vi "Actor Core.vi"(8 "error in":errorcluster, 11 "Generic Prompt in":refnum<class "Generic Prompt.lvclass">) -> (0 "Error Out":errorcluster, 3 "Actor out":refnum<class "Actor.lvclass">)   [LabVIEW 2014, in "Generic Prompt.lvlib" / "Generic Prompt.lvclass"]
doc: "(<B>Filename</B>: Actor Framework.lvlib:Actor.lvclass:Actor Core.vi)\n\nReceives messages to the actor, reacts to them, and initiates any error handling that may shut the actor down.\n\nDescendant classes may override this VI to append parallel tasks for the actor to complete while it handles messages. Overrides use the Call Parent Method node."
uses:
  Generic Prompt.lvclass
  <vilib>/ActorFramework/Actor/Actor.lvclass
  SetUp VIs/Instrument Finder/Instrument Finder.lvclass
  Subpanel Insertion/Subpanel Inserter.lvclass
  <vilib>/event_ctls.llb/eventsource.ctl
  <vilib>/event_ctls.llb/lveventtype.ctl
  <vilib>/ActorFramework/Message Enqueuer/Message Enqueuer.lvclass
  <vilib>/ActorFramework/Message Enqueuer/Message Enqueuer.lvclass/Message Enqueuer.ctl
  <vilib>/ActorFramework/Actor/Actor.lvclass/Actor.ctl
  Subpanel Inserter Messages/Insert Into Subpanel Msg/Insert Into Subpanel Msg.lvclass/Insert Into Subpanel Msg.ctl
  <vilib>/ActorFramework/Message Enqueuer/Message Priority.ctl
  New Session Class/New Session.lvclass
  <vilib>/ActorFramework/Message Enqueuer/Enqueue.vi
  <vilib>/ActorFramework/Message Enqueuer/Init from Existing Queue.vi
  <vilib>/ActorFramework/Message Priority Queue/Priority Enqueue.vi
  Subpanel Inserter Messages/Insert Into Subpanel Msg/Insert Into Subpanel Msg.lvclass
  <vilib>/ActorFramework/Stop Msg/Stop Msg.lvclass
  <vilib>/MGI/Monitored Actor/Actor/Monitored Actor.lvclass
panel:
  out "array address size":i32
  out "class name":string
  out "error out 4":errorcluster
  out "error out 3":errorcluster
  in  "cancel kid":bool
  out "Array of addresses":refnum<class "Message Enqueuer.lvclass">[](array[class])
  out "NewVal":bool
  out "OldVal":bool
  out "Time":u32
  out "Type":T1=enum."Value Change"
  out "Source":T2 items=["LabVIEW UI"=0, "ActiveX"=1, "User Event"=25]
  out "stopper":bool
  out "Array 2":string[](array[string])
  out "error out 2":errorcluster
  out "error out":errorcluster
  out "i- main":i32
  out "list of class":string[](array[string])
  out "Array Size":i32
  out "array size = counter? (next)":bool
  out "child to get":i32
  out "New Session SetUp is ON?":bool
  out "VI Name":string
  out "x = 0?":bool
  out "stop?":bool
  out "counter":i32
  out "i":i32
  in  "Array":refnum<class "Subpanel Inserter.lvclass">[](array[class])
  in  "SetUp VIs.lvlib:Instrument Finder.lvclass":refnum<class "Instrument Finder.lvclass">
  in  "Previous Button":bool
  in  "Next Button":bool
  in  "Stop Button":bool
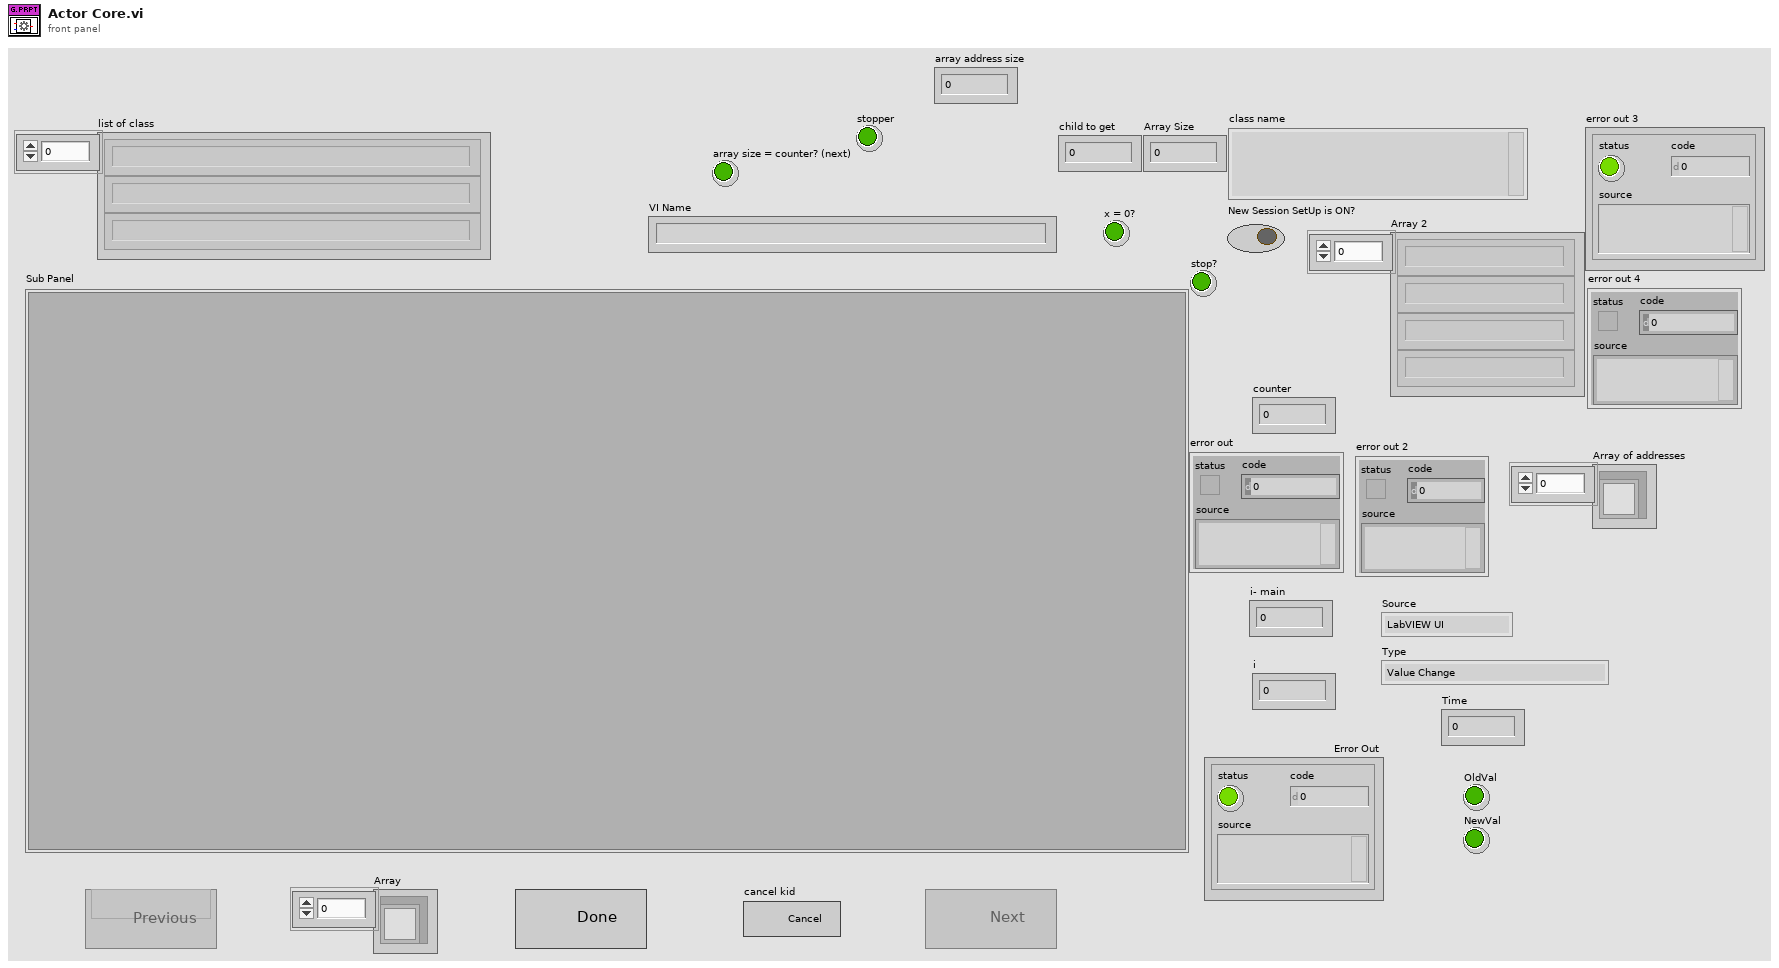
[diagram p1: front panel]
types:
  T1 = typedef "lveventtype.ctl" = enum32{"Null", "Timeout", "Annotation Menu Selection", "Annotation Menu Selection?", "App Instance Close", "App Instance Close?", "Autoscale Range Change", "Bookmark Info Change", "Cell Edit", "Cell Edit?", "Cursor Grab", "Cursor Grab?", "Cursor Menu Selection", "Cursor Menu Selection?", "Cursor Move", "Cursor Release", "Data Change", "Direction Change", "Display State Change", "Drag Ended", "Drag Enter", "Drag Leave", "Drag Over", "Drag Source Update", "Drag Starting", "Drag Starting?", "Drop", "Exec State Change", "Key Down", "Key Down?", "Key Repeat", "Key Repeat?", "Key Up", "Listbox Double Click", "Menu Activation?", "Menu Selection (App)", "Menu Selection? (App)", "Menu Selection (User)", "Mouse Down", "Mouse Down?", "Mouse Enter", "Mouse Leave", "Mouse Move", "Mouse Up", "Mouse Wheel", "NI Security User Change (App)", "Pane Size", "Panel Close", "Panel Close?", "Panel Resize", "Plot Attribute Change", "Scale Range Change", "Shortcut Menu Activation?", "Shortcut Menu Selection (App)", "Shortcut Menu Selection? (App)", "Shortcut Menu Selection (User)", "Tree Double Click", "Tree Drag", "Tree Drag?", "Tree Drop", "Tree Drop?", "Tree Item Close", "Tree Item Close?", "Tree Item Open", "Tree Item Open?", "User Event", "Value Change"}
  T2 = typedef "eventsource.ctl" = u32
  T3 = enum8{"Enabled", "Disabled", "Disabled and Grayed Out"}
  T4 = typedef "Actor Framework.lvlib/Message Enqueuer.lvclass/Message Priority.ctl" = enum16{"Low", "Normal", "High"}
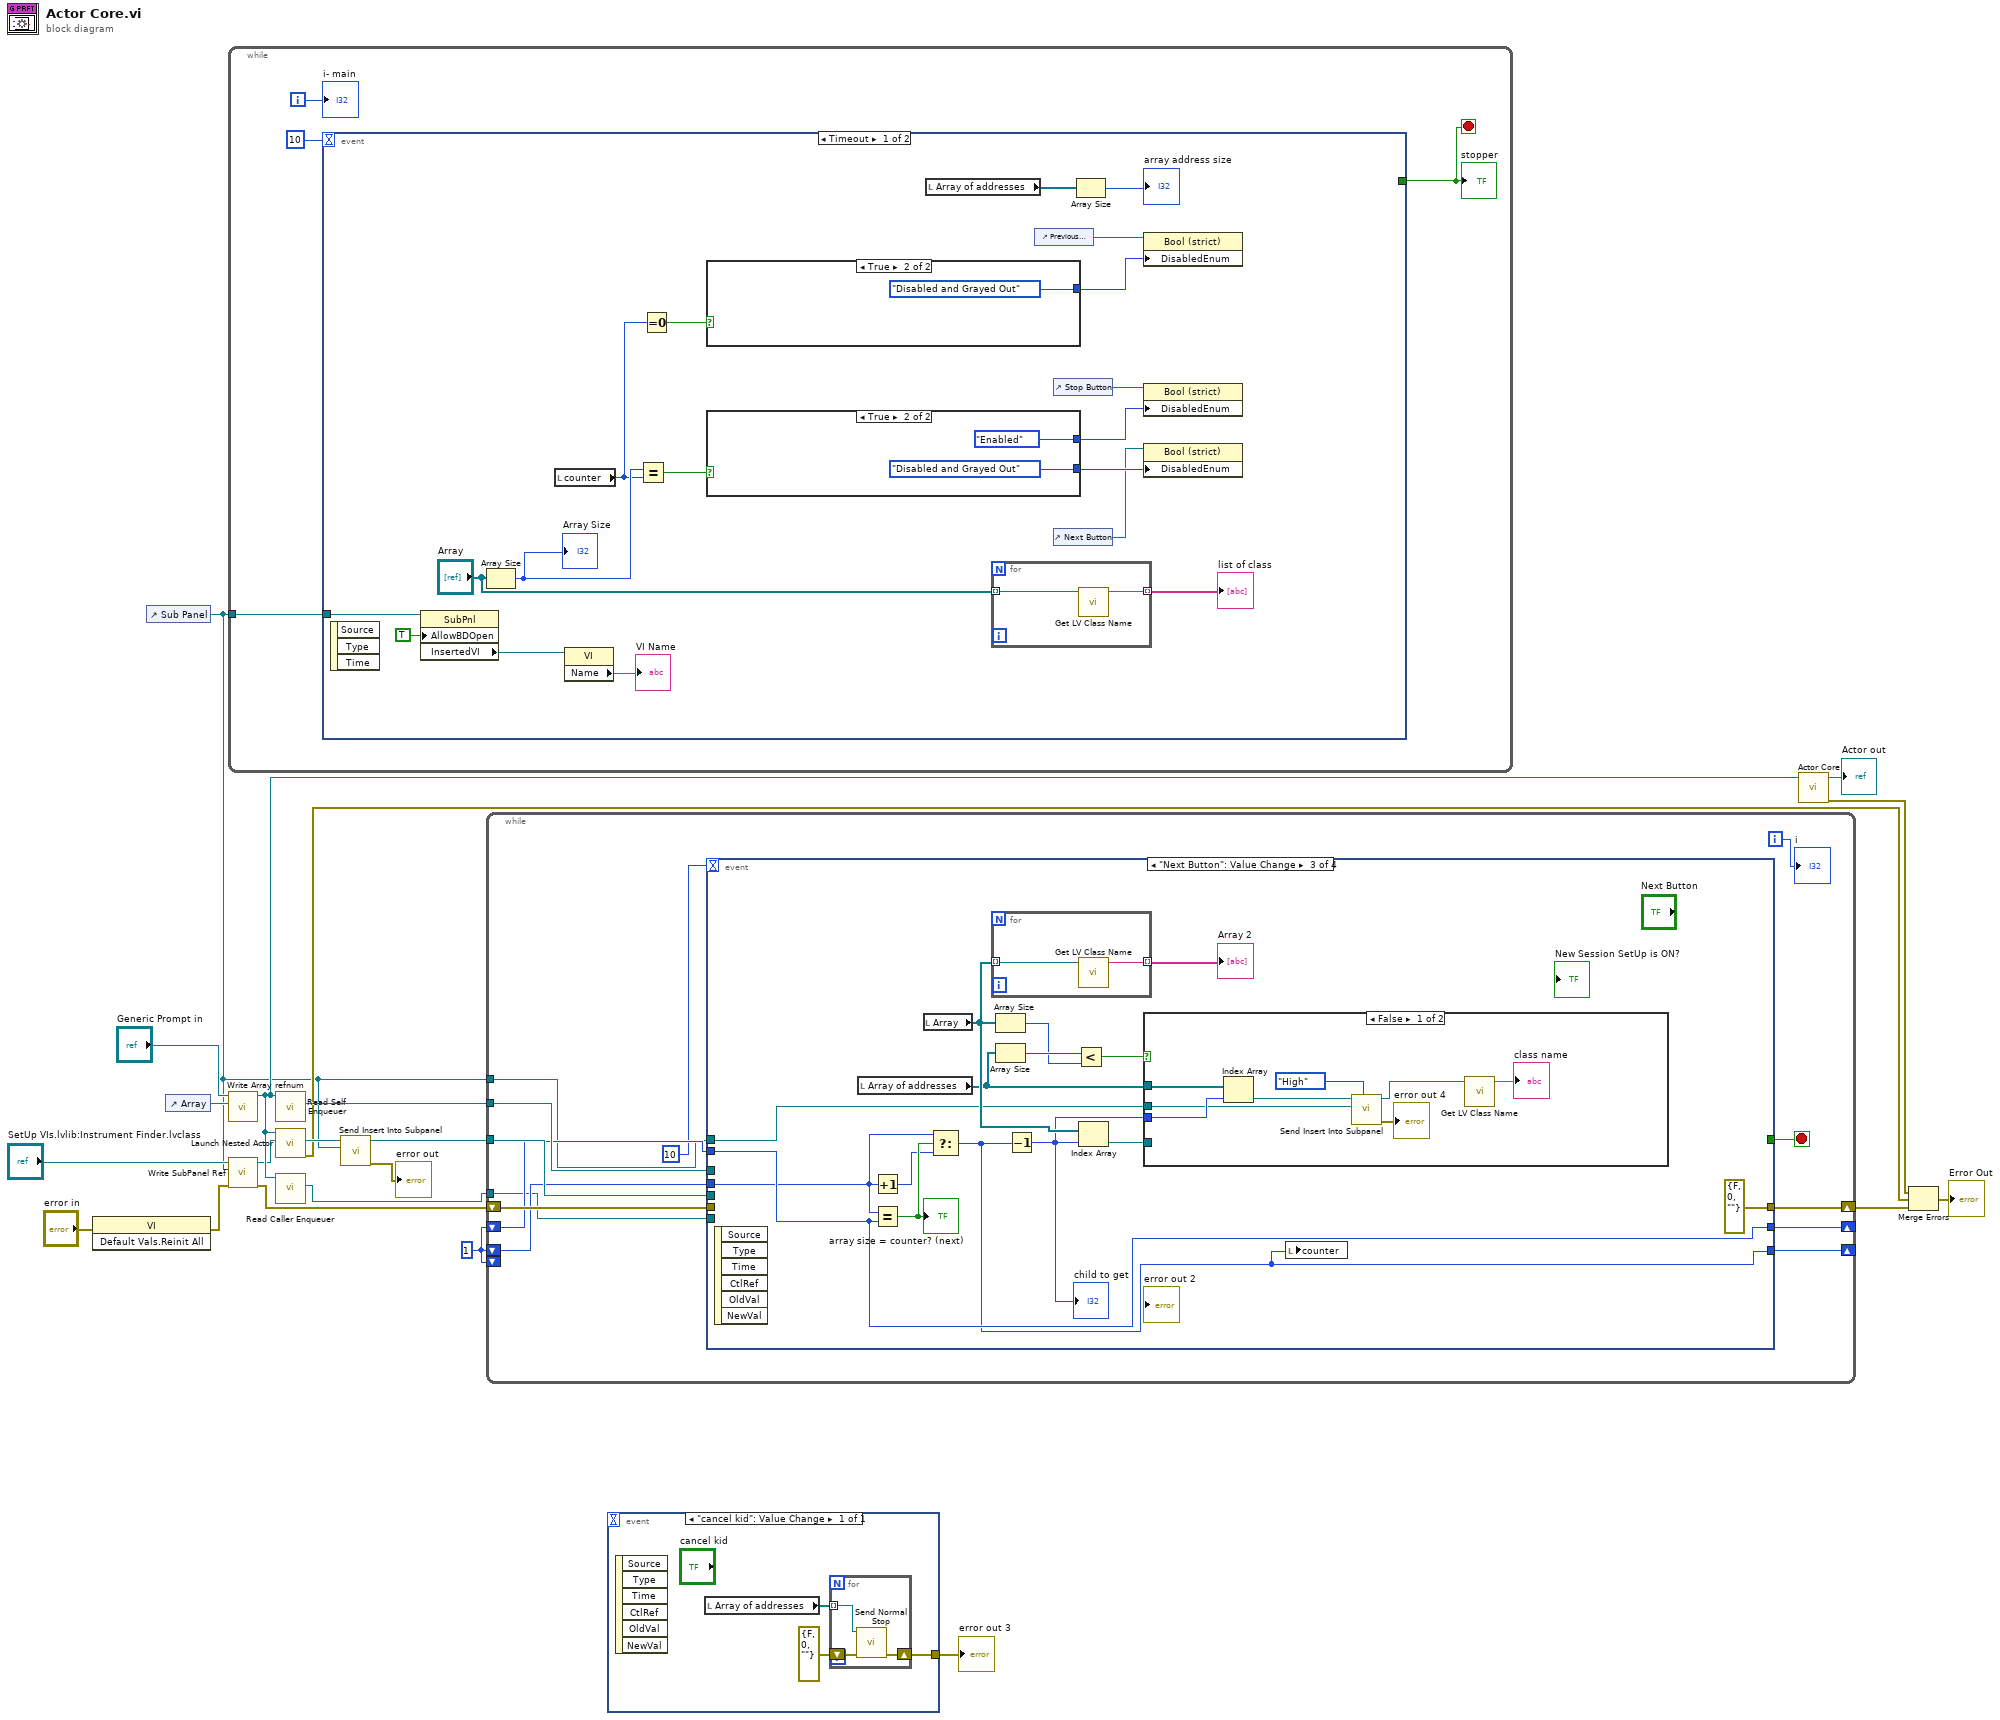
[diagram p0: block diagram]
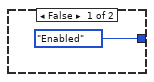
[diagram p2: hidden frame]
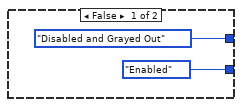
[diagram p3: hidden frame]
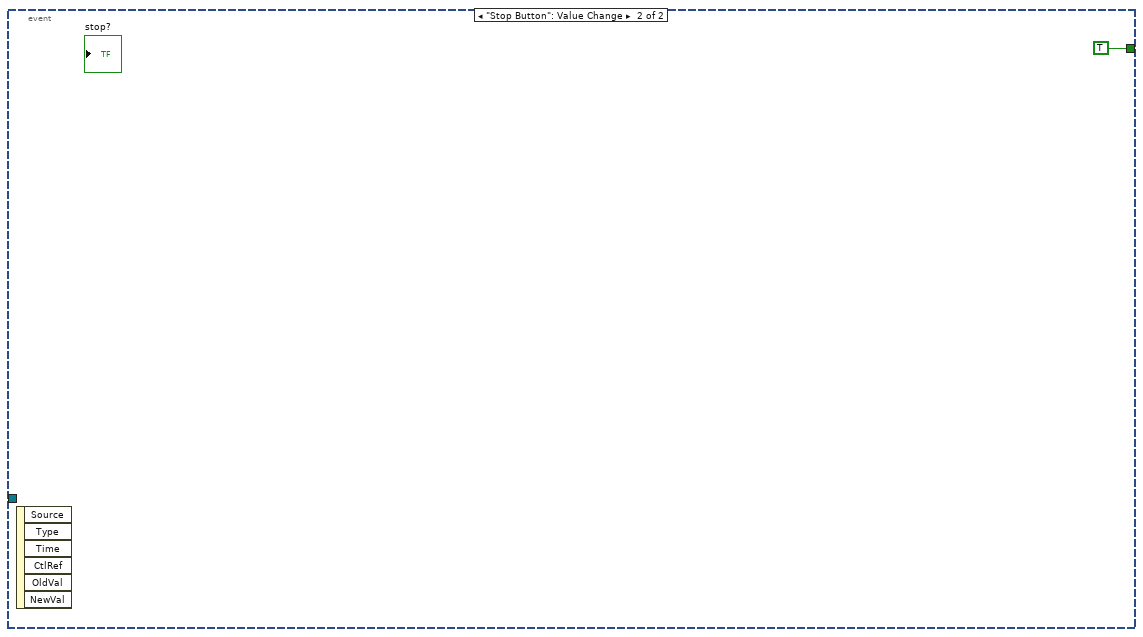
[diagram p4: hidden frame]
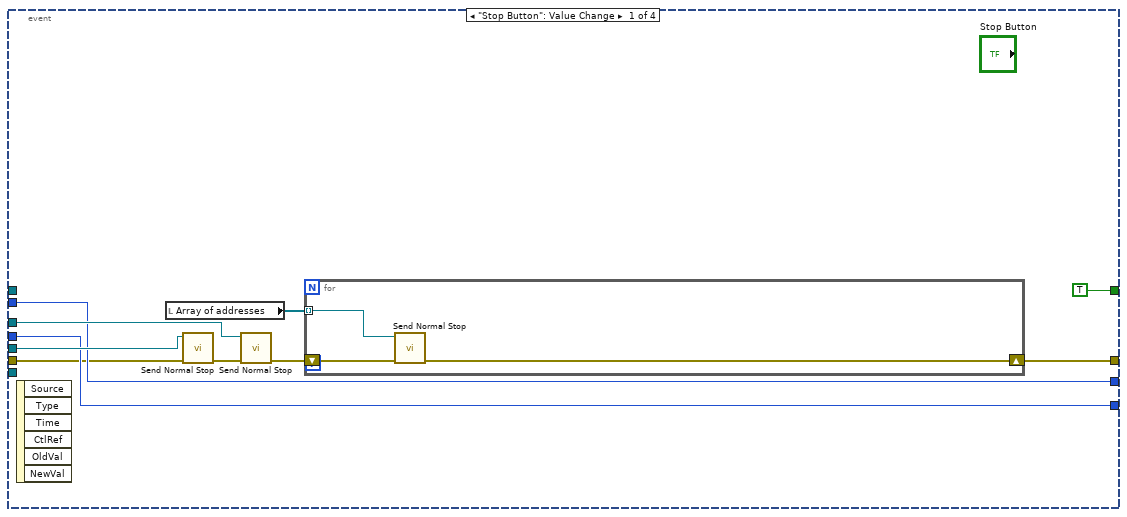
[diagram p5: hidden frame]
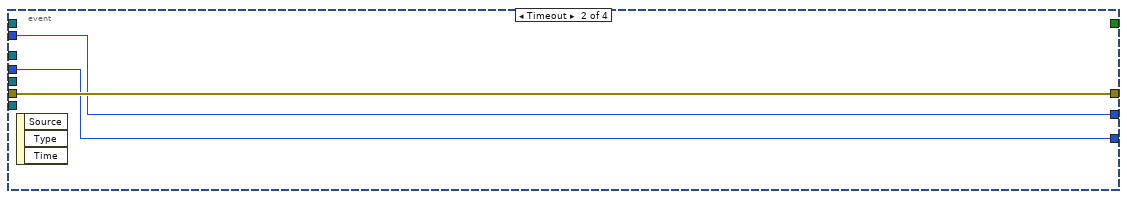
[diagram p6: hidden frame]
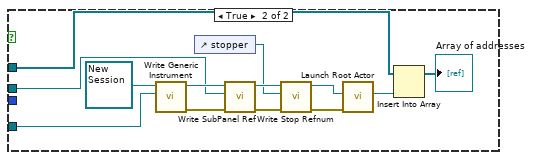
[diagram p7: hidden frame]
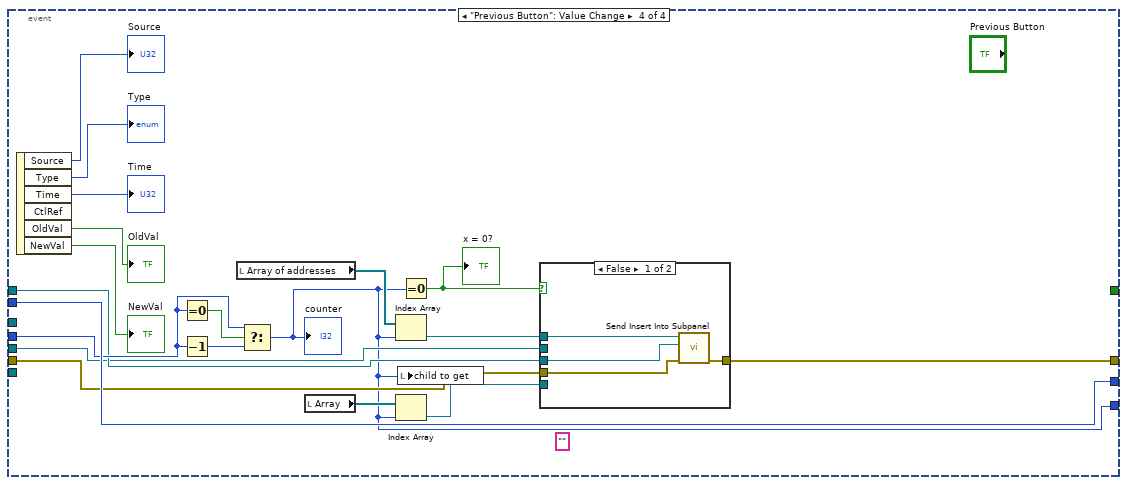
[diagram p8: hidden frame]
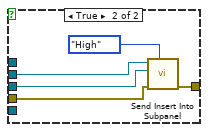
[diagram p9: hidden frame]
diagram:
  w17 = 1
  n1 = invoke class="VI" method="Default Vals.Reinit All"(error in="error in") -> (error out=w19:errorcluster)  [unwired: 2 in, 2 out]
  n2 = control-ref of="Sub Panel"() -> (w3:refnum<vi>)
  n3 = control-ref of="Array"() -> (w11:refnum<vi>)
  n4 = while {
    tunnel: w3 -> [w24]
    i -> [w22]
    stop <- w25 stop-if-true
    n5 = event shown="[0] Timeout" {
      selector: _ -> [_ _]
      dyn-events: _ -> [_ _]
      timeout: 10 -> [_ _]
      tunnel: [_ TRUE] -> w25
      tunnel: w24 -> [w35 _]
      event Timeout {
        n6 = event-data() -> ()  [unwired: 1 in, 3 out]
        n7 = property class="SubPnl"(reference=w35, "AllowBDOpen"=TRUE ("Allow User to Open Diagram")) -> ("InsertedVI"=w37:refnum<vi>)  [unwired: 1 in, 2 out]
        n8 = Array Size(array="Array") -> (size(s)=w31:i32)
        "Array Size" <- w31
        n9 = local read "counter"() -> (w28:i32)
        n10 = property class="VI"(reference=w37) -> ("Name"=→"VI Name":string)  [unwired: 1 in, 2 out]
        n11 = Equal?(x=w31, y=w28) -> (x = y?=w43:bool)
        n12 = Equal To 0?(x=w28) -> (x = 0?=w40:bool)
        n13 = case shown="True" w40 {
          tunnel: [T3."Enabled" ("Disabled") T3."Disabled and Grayed Out" ("Disabled")] -> w41
          frame False {
          }
          frame True {
          }
        }
        n14 = case shown="True" w43 {
          tunnel: [T3."Enabled" ("Disabled") T3."Disabled and Grayed Out" ("Disabled")] -> w42
          tunnel: [T3."Disabled and Grayed Out" ("Disabled") T3."Enabled" ("Disabled")] -> w39
          frame False {
          }
          frame True {
          }
        }
        n15 = local read "Array of addresses"() -> (w27:refnum<class "Message Enqueuer.lvclass">[])
        n16 = for {
          tunnel: "Array" -> [w45] mode=indexing
          tunnel: [w44] -> w29 mode=indexing
          n17 = call <vilib>:"Get LV Class Name.vi"("object"=w45) -> ("class name"=w44:string)  [unwired: 9 in, 1 out]
        }
        "list of class" <- w29
        n18 = control-ref of="Previous Button"() -> (w34:refnum<vi>)
        n19 = control-ref of="Stop Button"() -> (w32:refnum<vi>)
        n20 = control-ref of="Next Button"() -> (w33:refnum<vi>)
        n21 = Array Size(array=w27) -> (size(s)=→"array address size":i32)
        n22 = property on="Property Node" class="Bool (strict)"(reference=w34, "DisabledEnum"=w41) -> ()  [unwired: 1 in, 2 out]
        n23 = property on="Property Node" class="Bool (strict)"(reference=w32, "DisabledEnum"=w39) -> ()  [unwired: 1 in, 2 out]
        n24 = property on="Property Node" class="Bool (strict)"(reference=w33, "DisabledEnum"=w42) -> ()  [unwired: 1 in, 2 out]
      }
      event "Stop Button": Value Change {
        n25 = event-data() -> ()  [unwired: 1 in, 6 out]
      }
    }
    "stopper" <- w25
    "i- main" <- w22
  }
  n26 = call-dynamic "Write Array refnum.vi"("Array refnum"=w11, "Generic Prompt in"="Generic Prompt in") -> ("Generic Prompt out"=w15:refnum<class "Generic Prompt.lvclass">)  [unwired: 8 in, 1 out]
  n27 = call-dynamic "Write SubPanel Ref.vi"("error in (no error)"=w19, "SubPanel Ref"=w3, "Subpanel Inserter in"="SetUp VIs.lvlib:Instrument Finder.lvclass") -> ("error out"=w9:errorcluster, "Subpanel Inserter out"=w10:refnum<class "Instrument Finder.lvclass">)  [unwired: 7 in]
  n28 = call <vilib>:"Read Self Enqueuer.vi"("Actor"=w15) -> ("Self Enqueuer"=w16:refnum<class "Message Enqueuer.lvclass">)  [unwired: 10 in]
  n29 = call <vilib>:"Launch Nested Actor.vi"("Nested Actor"=w10, "Caller Actor in"=w15) -> ("error out"=w5:errorcluster, "Nested Actor's Enqueuer"=w7:refnum<class "Message Enqueuer.lvclass">)  [unwired: 7 in, 1 out]
  n30 = call <vilib>:"Read Caller Enqueuer.vi"("Actor"=w15) -> ("Caller Enqueuer"=w8:refnum<class "Message Enqueuer.lvclass">)  [unwired: 10 in]
  n31 = call "Send Insert Into Subpanel.vi"("SubPanel Ref"=w3, "Message Enqueuer"=w7) -> ("error out"=→"error out":errorcluster, "Message Enqueuer out"=w6:refnum<class "Message Enqueuer.lvclass">)  [unwired: 8 in]
  n32 = while {
    tunnel: w6 -> [w65]
    shift-right: [w62] -> w14
    shift-left: w9 -> [w63]
    tunnel: w16 -> [w61]
    shift-right: [w55] -> _
    shift-left: w17 -> [w56]
    shift-left: w17 -> [_]
    shift-right: [w58] -> _
    shift-left: w17 -> [w59]
    tunnel: w3 -> [w57]
    tunnel: w8 -> [w54]
    i -> [w60]
    stop <- w64 stop-if-true
    n33 = event shown="[2] \"Next Button\": Value Change" {
      selector: _ -> [_ _ _ _]
      dyn-events: _ -> [_ _ _ _]
      timeout: 10 -> [_ _ _ _]
      tunnel: w65 -> [w75 _ _ w129]
      tunnel: [TRUE _ _ _] -> w64
      tunnel: w63 -> [w69 w81 _ w134]
      tunnel: [w66 w81 errorcluster {"status"=FALSE, "code"=0, "source"=""} ("error out") w133] -> w62
      tunnel: w61 -> [w74 _ _ _]
      tunnel: w56 -> [w73 w79 w84 w136]
      tunnel: [w73 w79 w92 w121] -> w55
      tunnel: w59 -> [w72 w80 w96 w138]
      tunnel: [w72 w80 w96 w138] -> w58
      tunnel: w57 -> [_ _ w85 w132]
      tunnel: w54 -> [_ _ _ _]
      event "Stop Button": Value Change {
        n34 = event-data() -> ()  [unwired: 1 in, 6 out]
        n35 = local read "Array of addresses"() -> (w68:refnum<class "Message Enqueuer.lvclass">[])
        n36 = call <vilib>:"Send Normal Stop.vi"("error in (no error)"=w69, "Message Enqueuer"=w75) -> ("error out"=w70:errorcluster)  [unwired: 9 in]
        n37 = call <vilib>:"Send Normal Stop.vi"("error in (no error)"=w70, "Message Enqueuer"=w74) -> ("error out"=w67:errorcluster)  [unwired: 9 in]
        n38 = for {
          tunnel: w68 -> [w78] mode=indexing
          shift-right: [w77] -> w66
          shift-left: w67 -> [w76]
          n39 = call <vilib>:"Send Normal Stop.vi"("error in (no error)"=w76, "Message Enqueuer"=w78) -> ("error out"=w77:errorcluster)  [unwired: 9 in]
        }
      }
      event Timeout {
        n40 = event-data() -> ()  [unwired: 1 in, 3 out]
      }
      event "Next Button": Value Change {
        n41 = event-data() -> ()  [unwired: 1 in, 6 out]
        n42 = local read "Array of addresses"() -> (w83:refnum<class "Message Enqueuer.lvclass">[])
        n43 = Increment(x=w84) -> (x+1=w94:i32)
        n44 = Equal?(x=w84, y=w96) -> (x = y?=w95:bool)
        "array size = counter? (next)" <- w95
        n45 = local read "Array"() -> (w90:refnum<class "Subpanel Inserter.lvclass">[])
        n46 = Select(t=w84, s=w95, f=w94) -> (s? t:f=w92:i32)
        n47 = for {
          tunnel: w90 -> [w119] mode=indexing
          tunnel: [w118] -> w91 mode=indexing
          n48 = call <vilib>:"Get LV Class Name.vi"("object"=w119) -> ("class name"=w118:string)  [unwired: 9 in, 1 out]
        }
        "Array 2" <- w91
        n49 = Array Size(array=w90) -> (size(s)=w88:i32)
        n50 = Array Size(array=w83) -> (size(s)=w89:i32)
        n51 = Decrement(x=w92) -> (x-1=w82:i32)
        "child to get" <- w82
        n52 = Less?(x=w89, y=w88) -> (x < y?=w87:bool)
        n53 = Index Array(array=w90, index=w82) -> (element=w86:refnum<class "Subpanel Inserter.lvclass">)
        n54 = case shown="False" w87 {
          tunnel: w86 -> [_ w116]
          tunnel: w85 -> [w101 w113]
          tunnel: w83 -> [w104 w105]
          tunnel: w82 -> [w103 _]
          frame False {
            n55 = Index Array(array=w104, index=w103) -> (element=w102:refnum<class "Message Enqueuer.lvclass">)
            n56 = call "Send Insert Into Subpanel.vi"("Message Priority (Normal)"=Message_Priority."High", "SubPanel Ref"=w101, "Message Enqueuer"=w102) -> ("error out"=→"error out 4":errorcluster, "Message Enqueuer out"=w97:refnum<class "Message Enqueuer.lvclass">)  [unwired: 7 in]
            n57 = call <vilib>:"Get LV Class Name.vi"("object"=w97) -> ("class name"=→"class name":string)  [unwired: 9 in, 1 out]
          }
          frame True {
            n58 = call-dynamic "Write Generic Instrument.vi"("Subpanel Insertion.lvlib:Subpanel Inserter.lvclass"=w116, "New Session in"=refnum<class "New Session.lvclass"> refnum ("New Session Class.lvlib:New Session.lvclass")) -> ("error out"=w114:errorcluster, "New Session out"=w115:refnum<class "New Session.lvclass">)  [unwired: 8 in]
            n59 = control-ref of="stopper"() -> (w110:refnum<vi>)
            n60 = call-dynamic "Write SubPanel Ref.vi"("error in (no error)"=w114, "SubPanel Ref"=w113, "Subpanel Inserter in"=w115) -> ("error out"=w111:errorcluster, "Subpanel Inserter out"=w112:refnum<class "New Session.lvclass">)  [unwired: 7 in]
            n61 = call-dynamic "Write Stop Refnum.vi"("error in (no error)"=w111, "Stop Refnum"=w110, "New Session in"=w112) -> ("error out"=w108:errorcluster, "New Session out"=w109:refnum<class "New Session.lvclass">)  [unwired: 7 in]
            n62 = call <vilib>:"Launch Root Actor.vi"("error in (no error)"=w108, "Actor"=w109) -> ("Actor's Enqueuer"=w107:refnum<class "Message Enqueuer.lvclass">)  [unwired: 8 in, 1 out]
            n63 = Insert Into Array(array=w105, new element=w107) -> (→"Array of addresses":refnum<class "Message Enqueuer.lvclass">[])  [unwired: 1 in]
          }
        }
        n64 = local write "counter"(w92) -> ()
      }
      event "Previous Button": Value Change {
        (unwired) ""
        n65 = event-data() -> ("Source"=→"Source":T2, "Type"=→"Type":T1, "Time"=→"Time":u32, "OldVal"=→"OldVal":bool, "NewVal"=→"NewVal":bool)  [unwired: 1 in, 1 out]
        n66 = Equal To 0?(x=w136) -> (x = 0?=w131:bool)
        n67 = Decrement(x=w136) -> (x-1=w137:i32)
        n68 = local read "Array of addresses"() -> (w122:refnum<class "Message Enqueuer.lvclass">[])
        n69 = Select(t=w136, s=w131, f=w137) -> (s? t:f=w121:i32)
        "counter" <- w121
        n70 = local read "Array"() -> (w128:refnum<class "Subpanel Inserter.lvclass">[])
        n71 = Index Array(array=w122, index=w121) -> (element=w120:refnum<class "Message Enqueuer.lvclass">)
        n72 = Index Array(array=w128, index=w121) -> (element=w135:refnum<class "Subpanel Inserter.lvclass">)
        n73 = local write "child to get"(w121) -> ()
        n74 = Equal To 0?(x=w121) -> (x = 0?=w130:bool)
        "x = 0?" <- w130
        n75 = case shown="False" w130 {
          tunnel: w134 -> [w141 w147]
          tunnel: [w142 w146] -> w133
          tunnel: w132 -> [w140 w145]
          tunnel: w135 -> [_ _]
          tunnel: w129 -> [_ w143]
          tunnel: w120 -> [w139 _]
          frame False {
            n76 = call "Send Insert Into Subpanel.vi"("error in (no error)"=w141, "SubPanel Ref"=w140, "Message Enqueuer"=w139) -> ("error out"=w142:errorcluster)  [unwired: 7 in, 1 out]
          }
          frame True {
            n77 = call "Send Insert Into Subpanel.vi"("Message Priority (Normal)"=Message_Priority."High", "error in (no error)"=w147, "SubPanel Ref"=w145, "Message Enqueuer"=w143) -> ("error out"=w146:errorcluster)  [unwired: 6 in, 1 out]
          }
        }
      }
    }
    "i" <- w60
  }
  n78 = event shown="[0] \"cancel kid\": Value Change" {
    selector: _ -> [_]
    dyn-events: _ -> [_]
    timeout: _ -> [_]
    tunnel: [w149] -> w1
    event "cancel kid": Value Change {
      n79 = event-data() -> ()  [unwired: 1 in, 6 out]
      n80 = local read "Array of addresses"() -> (w150:refnum<class "Message Enqueuer.lvclass">[])
      n81 = for {
        tunnel: w150 -> [w153] mode=indexing
        shift-right: [w152] -> w149
        shift-left: errorcluster {"status"=FALSE, "code"=0, "source"=""} ("error out") -> [w151]
        n82 = call <vilib>:"Send Normal Stop.vi"("error in (no error)"=w151, "Message Enqueuer"=w153) -> ("error out"=w152:errorcluster)  [unwired: 9 in]
      }
    }
  }
  "error out 3" <- w1
  n83 = call-parent "Actor Core.vi"("Actor in"=w15) -> ("error out"=w4:errorcluster, "Actor out"=→"Actor out":refnum<class "Actor.lvclass">)  [unwired: 9 in]
  n84 = Merge Errors(w4, w5, w14) -> (→"Error Out":errorcluster)
